vi "Get AP Sx Sig Curve Val.vi"(0 "asicHandle":i32, 1 "yScale":dbl, 5 "xArray":dbl, 7 "yArray":dbl, 9 "numPoints":i32, 11 "error in (no error)":errorcluster caption="错误输入（无错误）") -> (4 "function return":i32, 6 "xArray out":dbl, 8 "yArray out":dbl, 10 "numPoints out":i32, 15 "error out":errorcluster caption="错误输出")   [LabVIEW 2018]
doc: "extern int __stdcall GetAPSxSigCurveVal (int asicHandle, OUT double ** xArray, OUT double ** yArray, OUT int * numPoints, IN double yScale);"
uses:
  APSx.dll/APSx.dll
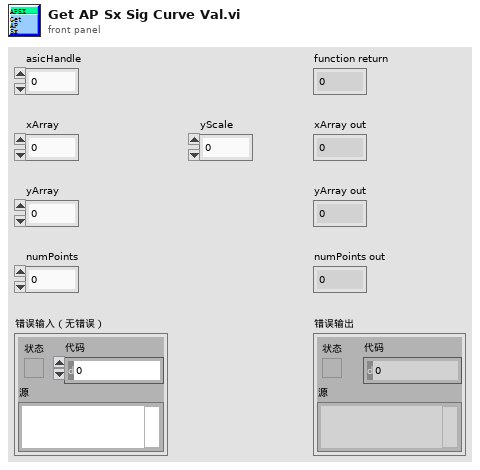
[diagram p1: front panel]
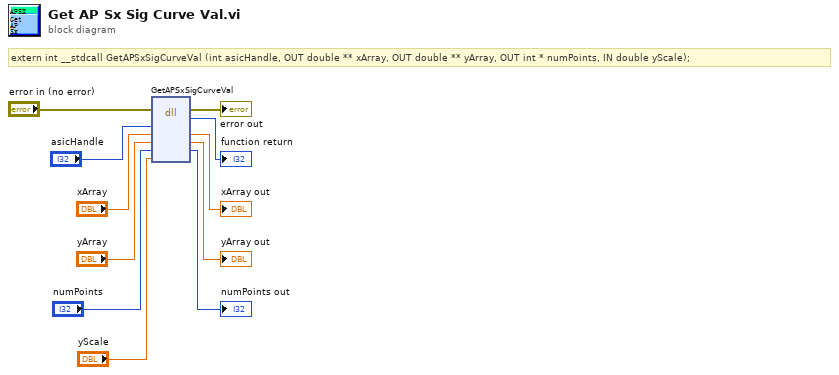
[diagram p0: block diagram]
diagram:
  # "extern int __stdcall GetAPSxSigCurveVal (int asicHandle, OUT double ** xArray, OUT double ** yArray, OUT int * numPoints, IN double yScale);"
  n1 = dll-call lib="PTH2[abs D项目Feng恒隆项目Labview传感器对中台SourcesAPSx.dllAPSx.*" fn="GetAPSxSigCurveVal"(error in="error in (no error)", "asicHandle"="asicHandle", "xArray"="xArray", "yArray"="yArray", "numPoints"="numPoints", "yScale"="yScale") -> (error out=→"error out":errorcluster, →"function return":i32, "xArray"=→"xArray out":dbl, "yArray"=→"yArray out":dbl, "numPoints"=→"numPoints out":i32)  [unwired: 4 in, 1 out]
